vi "DoLogoutUser.vi"(6 "error in (no error)":errorcluster, 9 "Sequence Context In":refnum<k7>) -> (0 "error out":errorcluster, 3 "Sequence Context Out":refnum<k7>)   [LabVIEW 2020]
doc: "Logout the Current TestStand User"
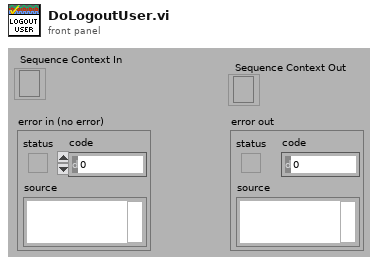
[diagram p1: front panel]
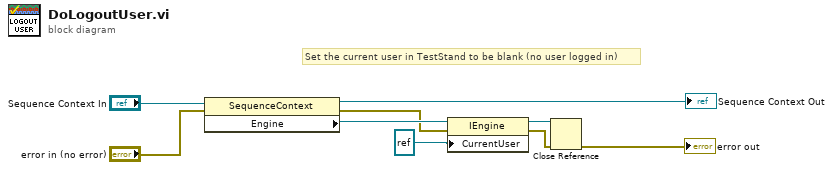
[diagram p0: block diagram]
diagram:
  # "Set the current user in TestStand to be blank (no user logged in)"
  n1 = property class="SequenceContext"(reference="Sequence Context In", error in="error in (no error)") -> (reference out=→"Sequence Context Out":refnum<k7>, error out=w3:errorcluster, "Engine"=w4:refnum<k7>)
  n2 = property class="IEngine"(reference=w4, error in=w3, "CurrentUser"=refnum<k7> refnum) -> (reference out=w7:refnum<k7>, error out=w6:errorcluster)
  n3 = Close Reference(reference=w7, error in (no error)=w6) -> (error out=→"error out":errorcluster)
